vi "NextState_TDMS.vi"(6 "end of file?":bool, 8 "error in (no error)":errorcluster, 10 "?":T1={"Start/End"=enum."Start", "stop"=FALSE, "file path"=path "", "OrderAnalysis"={"dB on"=TRUE, "window type"=1, "max order to analyze"=32.0, "order resolution"=0.1, "Axis"=0, "Sample rate"=5000, "Save?"=FALSE, "Multiple_Frequency"=3, "averaging mode"=enum."No averaging"}, "Meassurement Mode"={"Sample mode"=10123, "Terminal conf"=12529, "Channels"=""}} {"Meassurement Mode"."Terminal conf" items=["Default"=-1, "RSE"=10083, "NRSE"=10078, "Differential"=10106, "Pseudodifferential"=12529]; "Meassurement Mode"."Sample mode" items=["Finite Samples"=10178, "Continuous Samples"=10123, "Hardware Timed Single Point"=12522]; "OrderAnalysis"."Axis" items=["X", "Y", "Z"]; "OrderAnalysis"."window type" items=["No averaging", "Vector averaging", "RMS averaging", "Peak hold"]}, 11 "Previous Step":T6) -> (0 "error out":errorcluster, 3 "Next Step":T6)   [LabVIEW 2021]
uses:
  Typedefs/Stany.ctl
  Typedefs/PropertiesRead_TDM.ctl
  Typedefs/Start_End.ctl
  Typedefs/OrderAnalysis.ctl
  Typedefs/Axis.ctl
  Typedefs/MeassurementMode.ctl
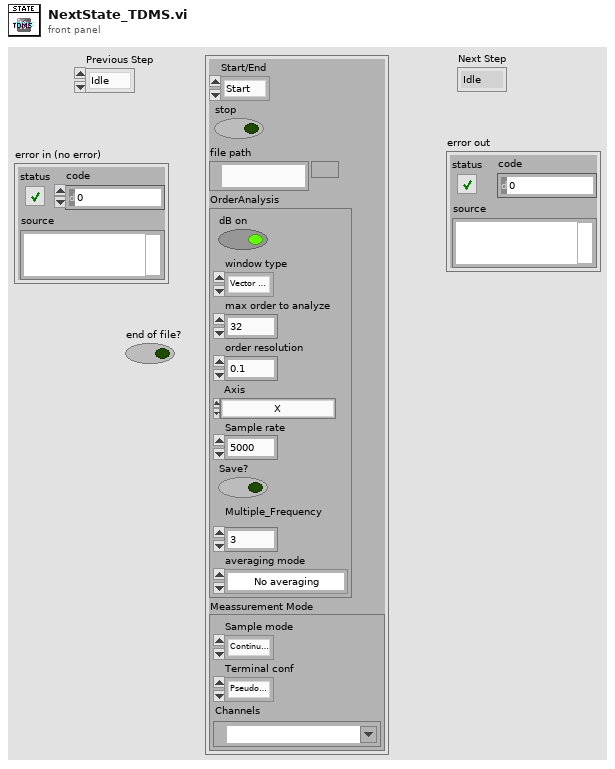
[diagram p1: front panel]
types:
  T1 = typedef "PropertiesRead_TDM.ctl" = cluster{"Start/End":T2, "stop":bool, "file path":path, "OrderAnalysis":T3, "Meassurement Mode":T5}
  T2 = typedef "Start_End.ctl" = enum16{"Start", "End"}
  T3 = typedef "OrderAnalysis.ctl" = cluster{"dB on":bool, "window type":u32, "max order to analyze":dbl, "order resolution":dbl, "Axis":T4, "Sample rate":i64, "Save?":bool, "Multiple_Frequency":i32, "averaging mode":enum16{"No averaging", "Vector averaging", "RMS averaging", "Peak hold"}}
  T4 = typedef "Axis.ctl" = u16
  T5 = typedef "MeassurementMode.ctl" = cluster{"Sample mode":i32, "Terminal conf":i32, "Channels":tag}
  T6 = typedef "Stany.ctl" = enum16{"Idle", "Init", "Acq", "End"}
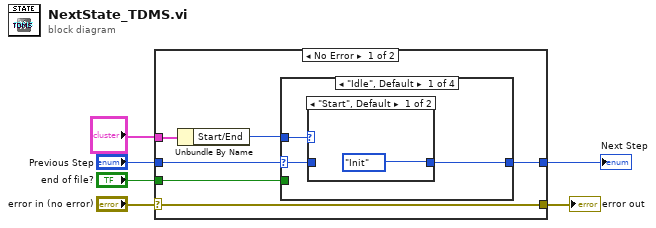
[diagram p0: block diagram]
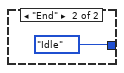
[diagram p2: hidden frame]
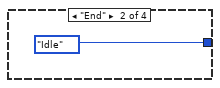
[diagram p3: hidden frame]
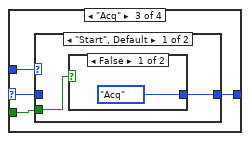
[diagram p4: hidden frame]
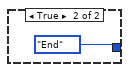
[diagram p5: hidden frame]
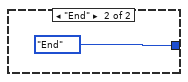
[diagram p6: hidden frame]
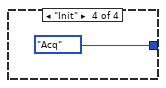
[diagram p7: hidden frame]
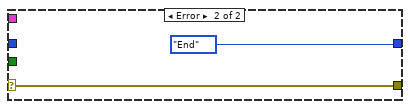
[diagram p8: hidden frame]
diagram:
  n1 = case shown="No Error" "error in (no error)" {
    selector: "error in (no error)" -> [w12 w30]
    tunnel: [w12 w30] -> w6
    tunnel: [w10 Stany."End" ("State")] -> w3
    tunnel: "?" -> [w9 _]
    tunnel: "Previous Step" -> [w11 _]
    tunnel: "end of file?" -> [w7 _]
    frame No Error {
      n2 = Unbundle By Name(w9) -> ("Start/End"=w8:T2)
      n3 = case shown="\"Idle\", Default" w11 {
        selector: w11 -> [w14 _ w21 _]
        tunnel: w8 -> [w15 _ w20 _]
        tunnel: [w13 Stany."Idle" ("State") w22 Stany."Acq" ("State")] -> w10
        tunnel: w7 -> [_ _ w19 _]
        frame "Idle", Default {
          n4 = case shown="\"Start\", Default" w15 {
            tunnel: [Stany."Init" ("State") Stany."Idle" ("State")] -> w13
            tunnel: w14 -> [_ _]
            frame "Start", Default {
            }
            frame "End" {
            }
          }
        }
        frame "End" {
        }
        frame "Acq" {
          n5 = case shown="\"Start\", Default" w20 {
            tunnel: [w24 Stany."End" ("State")] -> w22
            tunnel: w21 -> [_ _]
            tunnel: w19 -> [w23 _]
            frame "Start", Default {
              n6 = case shown="False" w23 {
                tunnel: [Stany."Acq" ("State") Stany."End" ("State")] -> w24
                frame False {
                }
                frame True {
                }
              }
            }
            frame "End" {
            }
          }
        }
        frame "Init" {
        }
      }
    }
    frame Error {
    }
  }
  "error out" <- w6
  "Next Step" <- w3
